vi "未命名 7.vi"() -> ()   [LabVIEW 2020]
panel:
  out "范围内？":bool[](array[boolean])
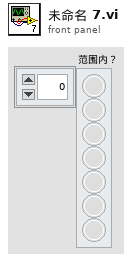
[diagram p1: front panel]
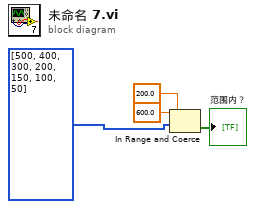
[diagram p0: block diagram]
diagram:
  n1 = In Range and Coerce(upper limit=600.0 ("上限"), x=i32[] [500, 400, 300, 200, 150, 100, 50], lower limit=200.0 ("下限")) -> (In Range?=→"范围内？":bool[])  [unwired: 1 out]
